vi "create Packet.vi"(8 "error in (no error)":errorcluster, 10 "Packet Type":T1, 11 "Packet in":refnum<class "Packet.lvclass">) -> (0 "error out":errorcluster, 3 "Packet out":refnum<class "Packet.lvclass">)   [LabVIEW 2019, in "Packet.lvclass"]
uses:
  Packet.lvclass
  packet type STYP.ctl
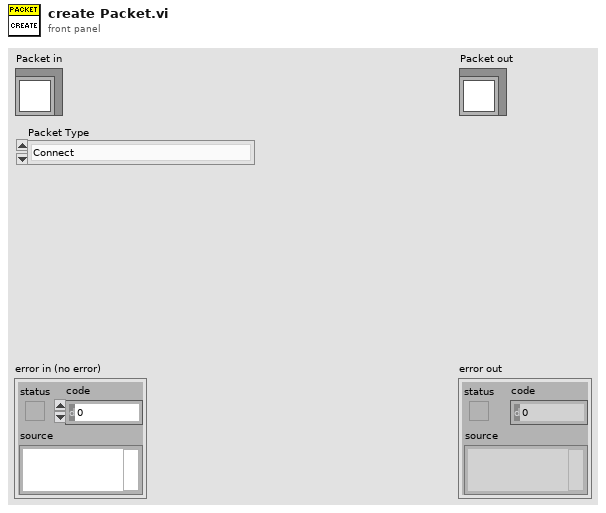
[diagram p1: front panel]
types:
  T1 = typedef "Packet.lvclass/packet type STYP.ctl" = enum16{"Connect", "Disconnect", "Direction", "Score", "Map"}
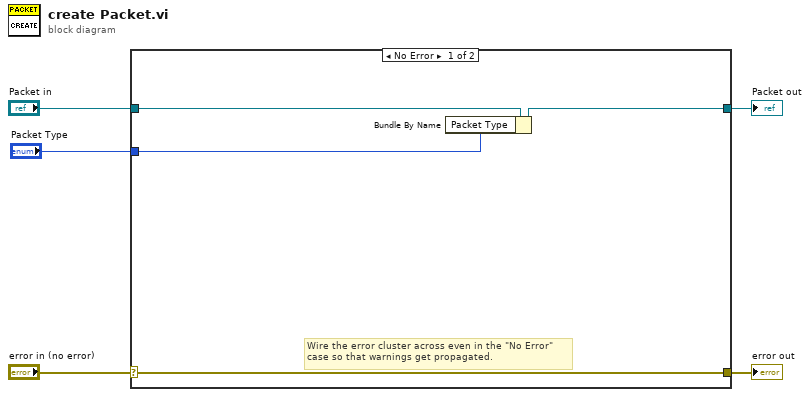
[diagram p0: block diagram]
diagram:
  n1 = case shown="No Error" "error in (no error)" {
    selector: "error in (no error)" -> [w8 w11]
    tunnel: [w8 w11] -> w4
    tunnel: [w7 w10] -> w2
    tunnel: "Packet in" -> [w9 w10]
    tunnel: "Packet Type" -> [w6 _]
    frame No Error {
      # "Wire the error cluster across even in the \"No Error\"\ncase so that warnings get propagated."
      n2 = Bundle By Name(cluster=w9, "Packet Type"=w6) -> (w7:refnum<class "Packet.lvclass">)
    }
    frame Error {
    }
  }
  "error out" <- w4
  "Packet out" <- w2
